vi "Stop Core.vi"(10 "final error code":i32, 11 "Line Tracker in":refnum<class "Line Tracker.lvclass">) -> (3 "Line Tracker out":refnum<class "Line Tracker.lvclass">)   [LabVIEW 2026, in "Line Tracker.lvlib" / "Line Tracker.lvclass"]
doc: "<p>(<strong>Filename</strong>: <span class=\"dnl\">Actor Framework.lvlib:Actor.lvclass:Stop Core.vi</span>)</p>\n<p>Defines what the actor does before it stops. Use the <strong>final error code</strong> input to determine whether the actor shut down in response to an error.</p>\n<p>By default, this method passes the Stop message along to all <a href=\"nihelplauncher://docs/csh?context=lvcore_lvcomm_af_launch_nested_actor\">auto-stop nested actors</a>. A descendant class may override this method to define additional behavior, such as shutting down any processes the actor initiated in its override of the <a href=\"nihelplauncher://docs/csh?context=lvcore_lvcomm_af_actor_core\">Actor Core</a> method.</p>"
uses:
  Line Tracker.lvclass
  <vilib>/ActorFramework/Actor/Actor.lvclass
  Line Tracker.lvclass/Line Tracker.ctl
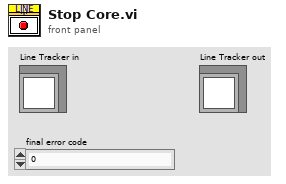
[diagram p1: front panel]
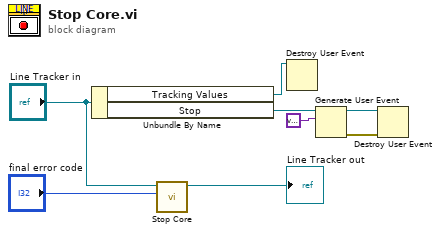
[diagram p0: block diagram]
diagram:
  n1 = Unbundle By Name("Line Tracker in") -> ("Tracking Values"=w1:refnum<user-event>, "Stop"=w5:refnum<user-event>)
  n2 = call-parent "Stop Core.vi"("final error code"="final error code", "Actor in"="Line Tracker in") -> ("Actor out"=→"Line Tracker out":refnum<class "Line Tracker.lvclass">)  [unwired: 9 in]
  n3 = Destroy User Event(user event=w1) -> ()  [unwired: 1 in, 1 out]
  n4 = Generate User Event(user event=w5, event data cluster=variant ("event data")) -> (user event out=w2:refnum<user-event>, error out=w3:errorcluster)  [unwired: 2 in]
  n5 = Destroy User Event(user event=w2, error in=w3) -> ()  [unwired: 1 out]
